vi "comm enable event.vi"(8 "error in (no error)":errorcluster, 10 "event mask":u32, 11 "Comm Handle":u64) -> (0 "error out":errorcluster, 3 "dup Comm Handle":u64)   [LabVIEW 2021, in "lvserial.lvlib"]
doc: "Specifies a set of events to be monitored for a communications device."
uses:
  lvserial.lvlib
  lvserial.dll
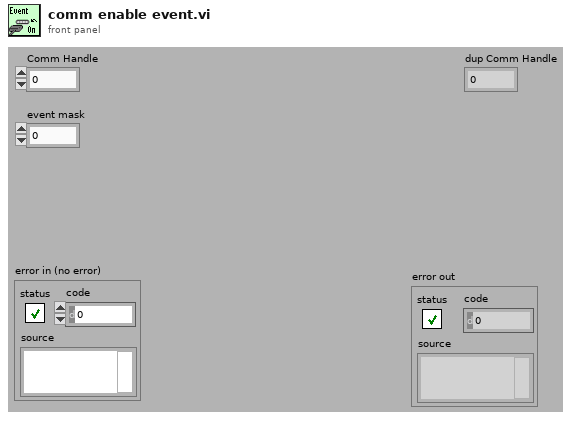
[diagram p1: front panel]
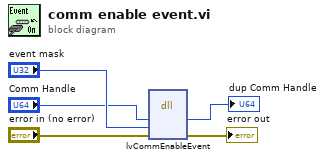
[diagram p0: block diagram]
diagram:
  n1 = dll-call lib="lvserial.dll" fn="lvCommEnableEvent"("hComm"="Comm Handle", "ulEventMask"="event mask", "error"="error in (no error)") -> ("hComm"=→"dup Comm Handle":u64, "error"=→"error out":errorcluster)  [unwired: 4 in, 3 out]
